vi "defaultTestResult.vi"(8 "error in (no error)":errorcluster, 10 "resultStatusChangedEventRef":refnum<user-event>, 11 "TestCase in":refnum<class "TestCase.lvclass">) -> (0 "error out":errorcluster, 2 "TestResult":refnum<class "TestResult.lvclass">, 3 "TestCase out":refnum<class "TestCase.lvclass">)   [LabVIEW 2011, in "TestCase.lvclass"]
uses:
  TestCase.lvclass
  TestResult/TestResult.lvclass
  TestResult/resultStatusChanged--Cluster.ctl
  TestResult/resultStatus--enum.ctl
panel:
  # "JKI VI Tester for LabVIEW\nhttp://jkisoft.com/vi-tester\nCopyright (C) 2007-2009, JKI <info@jkisoft.com>\nALL RIGHTS RESERVED"
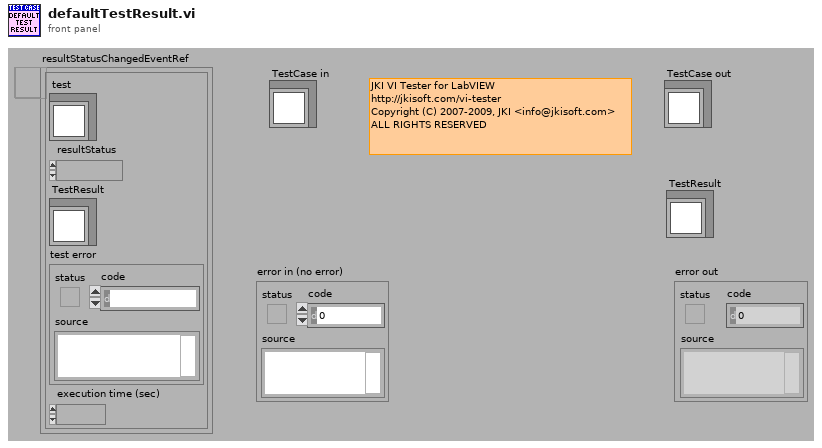
[diagram p1: front panel]
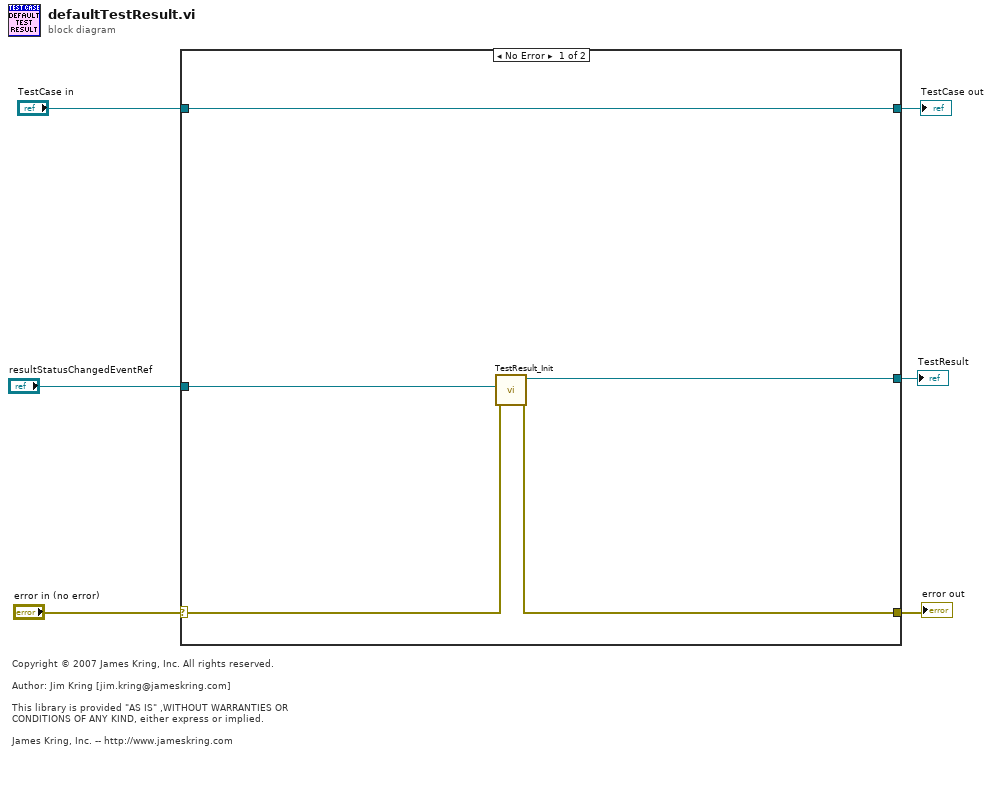
[diagram p0: block diagram]
diagram:
  # "Copyright © 2007 James Kring, Inc. All rights reserved.\n\nAuthor: Jim Kring [jim.kring@jameskring.com]\n\nThis library is provided \"AS IS\" ,WITHOUT WARRANTIES OR \nCONDITIONS OF ANY KIND, either express or implied.\n\nJames Kring, Inc. -- http://www.jameskring.com"
  n1 = case shown="No Error" "error in (no error)" {
    selector: "error in (no error)" -> [w9 w13]
    tunnel: [w8 w13] -> w5
    tunnel: [w11 w12] -> w3
    tunnel: "TestCase in" -> [w11 w12]
    tunnel: [w10 _] -> w2
    tunnel: "resultStatusChangedEventRef" -> [w7 _]
    frame No Error {
      n2 = call "TestResult_Init.vi"("error in (no error)"=w9, "resultStatusChangedEventRef"=w7) -> ("error out"=w8:errorcluster, "TestResult out"=w10:refnum<class "TestResult.lvclass">)  [unwired: 8 in]
    }
    frame Error {
    }
  }
  "error out" <- w5
  "TestCase out" <- w3
  "TestResult" <- w2
